vi "LibXML_ParseDoc.vi"(8 "error in":errorcluster, 11 "XML string":string) -> (0 "error out":errorcluster, 3 "doc":u32)   [LabVIEW 2019, in "Tools.lvlib" / "LibXML.lvlib"]
doc: "Loads the XML-file into memory.\nWhen using \"Assign schema\" the Schema-Cluster should be filled in, the schema referred to inside the xml file will be overruled. This way one can be sure that the right (your) xsd is used for validation.\nSchemalocation should hold the exact schemalocation; The namespac- uri should be the same as used in the xml-file. Prefix is not used here."
uses:
  LibXML.lvlib
  <vilib>/Utility/error.llb/Trim Whitespace.vi
  Tools.lvlib
  dll/libxml2.dll
panel:
  # "This software is FREE licensed under the GNU Lesser General Public License (see license.txt)."
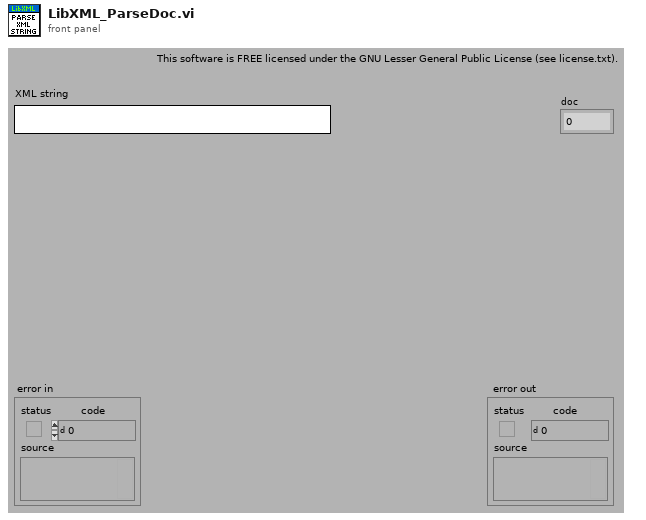
[diagram p1: front panel]
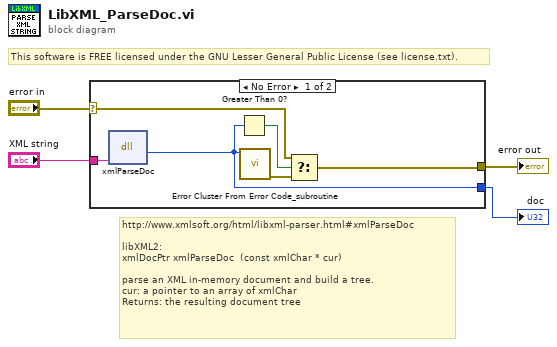
[diagram p0: block diagram]
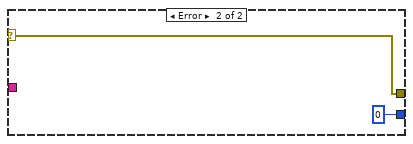
[diagram p2: hidden frame]
diagram:
  # "This software is FREE licensed under the GNU Lesser General Public License (see license.txt)."
  # "http://www.xmlsoft.org/html/libxml-parser.html#xmlParseDoc\n\nlibXML2:\nxmlDocPtr\txmlParseDoc\t\t(const xmlChar * cur)\n\nparse an XML in-memory document and build a tree.\ncur:\ta pointer to an array of xmlChar\nReturns:\tthe resulting document tree"
  n1 = case shown="No Error" "error in" {
    selector: "error in" -> [w5 w12]
    tunnel: [w8 w12] -> w4
    tunnel: [w7 u32 0] -> w2
    tunnel: "XML string" -> [w6 _]
    frame No Error {
      n2 = dll-call lib="C:/Projects/_Prywatne/MyCIT/Framework/Tools/XML/LibXML/dll/libxml2.dll" fn="xmlParseDoc"("XMLstring"=w6) -> ("return type"=w7:u32)  [unwired: 4 in, 2 out]
      n3 = Greater Than 0?(x=w7) -> (x > 0?=w10:bool)
      n4 = call "Error Cluster From Error Code_subroutine.vi"("error code (0)"=w7) -> ("error out"=w9:errorcluster)  [unwired: 8 in]
      n5 = Select(t=w5, s=w10, f=w9) -> (s? t:f=w8:errorcluster)
    }
    frame Error {
    }
  }
  "error out" <- w4
  "doc" <- w2
